vi "Example_digital_srq_wait.vi"() -> ()   [LabVIEW 2022 SP3]
uses:
  <vilib>/Instr/_visa.llb/Select Event Type.ctl
  usbtmc_scpi_labtool.lvlib
panel:
  out "status byte":u16
  in  "timeout (5000 ms)":u32=5000
  in  "VISA resource name in":refnum<visa-resource-name>="USB0::0xCAFE::0x4000::123456::INSTR"
  # "drive DIGI:INP2 low within the timeout"
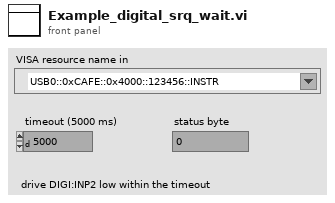
[diagram p1: front panel]
types:
  T1 = typedef "Select Event Type.ctl" = u32
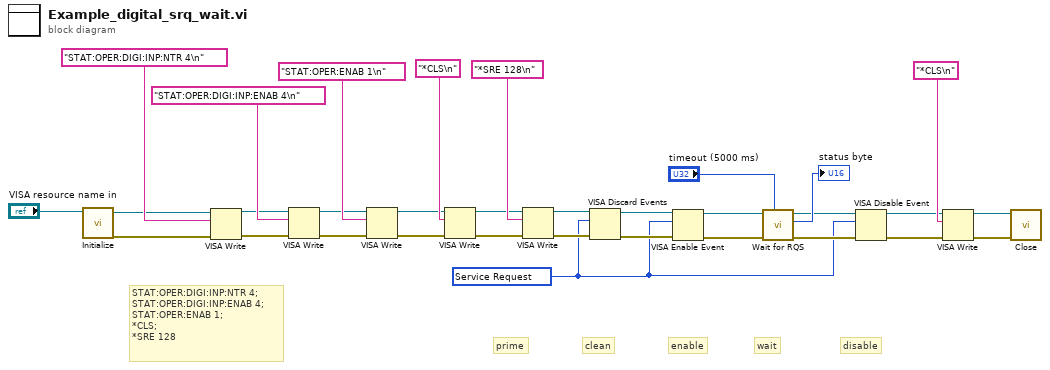
[diagram p0: block diagram]
diagram:
  w20 = T1 1073684491 items=["Service Request"=1073684491, "Trigger"=3221168138, "Clear"=1073684493, "VXI Signal"=1073684512, "VXI/VME Interrupt"=3221168161, "VXI/VME Sysfail"=1073684509, "VXI/VME Sysreset"=1073684510, "GPIB CIC"=1073684498, "GPIB Talk"=1073684499, "GPIB Listen"=1073684500, "PXI Interrupt"=1073684514, "Serial Break"=1073684515, "Serial TermChar"=1073684516, "Serial CTS"=1073684521, "Serial DSR"=1073684522, "Serial DCD"=1073684524, "Serial RI"=1073684526, "Serial Character"=1073684533, "USB Interrupt"=1073684535, "All Enabled"=1073709055] ("Event Type")
  # "disable"
  # "wait"
  # "prime"
  # "enable"
  # "clean"
  # "STAT:OPER:DIGI:INP:NTR 4;\nSTAT:OPER:DIGI:INP:ENAB 4;\nSTAT:OPER:ENAB 1;\n*CLS;\n*SRE 128"
  n1 = call "Initialize.vi"("VISA resource name in"="VISA resource name in") -> ("error out"=w8:errorcluster, "VISA resource name out"=w9:refnum<visa-resource-name>)  [unwired: 9 in]
  n2 = VISA Write(VISA resource name=w9, write buffer="STAT:OPER:DIGI:INP:NTR 4\n", error in (no error)=w8) -> (VISA resource name out=w7:refnum<visa-resource-name>, error out=w6:errorcluster)  [unwired: 1 out]
  n3 = VISA Write(VISA resource name=w7, write buffer="STAT:OPER:DIGI:INP:ENAB 4\n", error in (no error)=w6) -> (VISA resource name out=w13:refnum<visa-resource-name>, error out=w16:errorcluster)  [unwired: 1 out]
  n4 = VISA Write(VISA resource name=w13, write buffer="STAT:OPER:ENAB 1\n", error in (no error)=w16) -> (VISA resource name out=w12:refnum<visa-resource-name>, error out=w15:errorcluster)  [unwired: 1 out]
  n5 = VISA Write(VISA resource name=w12, write buffer="*CLS\n", error in (no error)=w15) -> (VISA resource name out=w11:refnum<visa-resource-name>, error out=w14:errorcluster)  [unwired: 1 out]
  n6 = VISA Write(VISA resource name=w11, write buffer="*SRE 128\n", error in (no error)=w14) -> (VISA resource name out=w30:refnum<visa-resource-name>, error out=w29:errorcluster)  [unwired: 1 out]
  n7 = VISA Discard Events(8:w29, 10:w20, 11:w30) -> (0:w27:errorcluster, 3:w28:refnum<visa-resource-name>)  [unwired: 1 in]
  n8 = VISA Enable Event(8:w27, 10:w20, 11:w28) -> (0:w25:errorcluster, 3:w26:refnum<visa-resource-name>)  [unwired: 1 in]
  n9 = call <vilib>:"Wait for RQS.vi"("timeout (25000 ms)"="timeout (5000 ms)", "error in (no error)"=w25, "VISA resource name"=w26) -> ("error out"=w21:errorcluster, "status byte"=→"status byte":u16, "VISA resource name out"=w22:refnum<visa-resource-name>)  [unwired: 6 in]
  n10 = VISA Disable Event(8:w21, 10:w20, 11:w22) -> (0:w3:errorcluster, 3:w4:refnum<visa-resource-name>)  [unwired: 1 in]
  n11 = VISA Write(VISA resource name=w4, write buffer="*CLS\n", error in (no error)=w3) -> (VISA resource name out=w2:refnum<visa-resource-name>, error out=w1:errorcluster)  [unwired: 1 out]
  n12 = call "Close.vi"("error in (no error)"=w1, "VISA resource name"=w2) -> ()  [unwired: 10 in]
